vi "Debug Ethernet Comms.vi"() -> ()   [LabVIEW 2021]
uses:
  Ethernet/Ethernet_BS1201.lvclass
panel:
  in  "Send RST":bool
  in  "Send Op Cfg":bool
  in  "stop":bool
  in  "Calibration Mode":bool
  in  "PID Disable":bool
  in  "Precision Mode":bool
  in  "UDP port":u16=54321
  in  "TCP port":u16=12345
  in  "Box IP address":string="192.168.1.100"
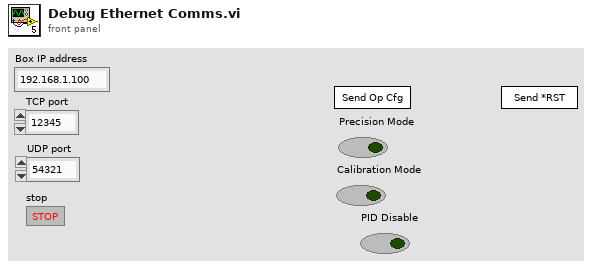
[diagram p1: front panel]
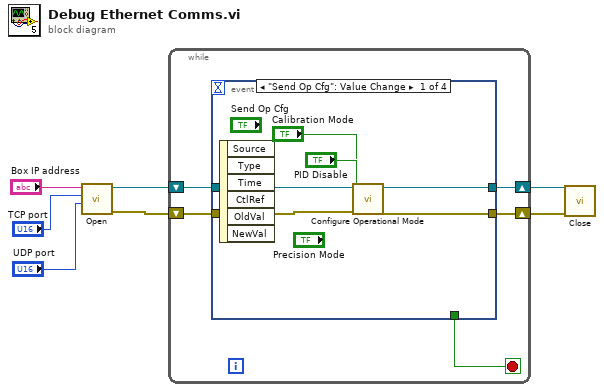
[diagram p0: block diagram]
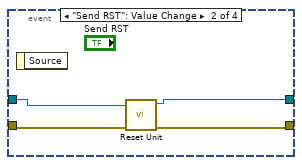
[diagram p2: hidden frame]
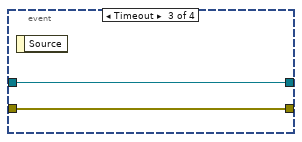
[diagram p3: hidden frame]
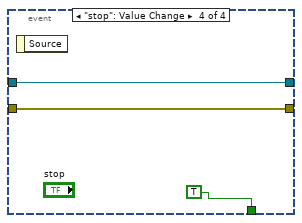
[diagram p4: hidden frame]
diagram:
  n1 = call "Open.vi"("UDP port"="UDP port", "TCP port"="TCP port", "Box IP address"="Box IP address") -> ("error out"=w3:errorcluster, "ENET out"=w4:refnum<class "Ethernet_BS1201.lvclass">)  [unwired: 7 in]
  n2 = while {
    shift-right: [w10] -> w2
    shift-left: w4 -> [w12]
    shift-right: [w9] -> w1
    shift-left: w3 -> [w11]
    stop <- w8 stop-if-true
    n3 = event shown="[0] \"Send Op Cfg\": Value Change" {
      selector: _ -> [_ _ _ _]
      dyn-events: _ -> [_ _ _ _]
      timeout: _ -> [_ _ _ _]
      tunnel: w12 -> [w18 w22 w24 w26]
      tunnel: w11 -> [w17 w19 w23 w25]
      tunnel: [w16 w21 w24 w26] -> w10
      tunnel: [w15 w20 w23 w25] -> w9
      tunnel: [_ _ _ TRUE] -> w8
      event "Send Op Cfg": Value Change {
        n4 = event-data() -> ()  [unwired: 1 in, 6 out]
        n5 = call-dynamic "Configure Operational Mode.vi"("error in (no error)"=w17, "Precision Mode"="PID Disable", "PID Disable"="Calibration Mode", "Ethernet in"=w18) -> ("error out"=w15:errorcluster, "Ethernet out"=w16:refnum<class "Ethernet_BS1201.lvclass">)  [unwired: 6 in]
      }
      event "Send RST": Value Change {
        n6 = event-data() -> ()  [unwired: 1 in, 1 out]
        n7 = call-dynamic "Reset Unit.vi"("error in (no error)"=w19, "Ethernet in"=w22) -> ("error out"=w20:errorcluster, "Ethernet out"=w21:refnum<class "Ethernet_BS1201.lvclass">)  [unwired: 8 in]
      }
      event Timeout {
        n8 = event-data() -> ()  [unwired: 1 in, 1 out]
      }
      event "stop": Value Change {
        n9 = event-data() -> ()  [unwired: 1 in, 1 out]
      }
    }
  }
  n10 = call-dynamic "Close.vi"("error in (no error)"=w1, "ENET in"=w2) -> ()  [unwired: 9 in, 1 out]
